vi "Write Websocket Data.vi"(6 "timeout ms (5000)":i32=500, 7 "Websocket Client Handler in":refnum<class "Websocket Client Handler.lvclass">, 8 "error in (no error)":errorcluster, 11 "Data":string) -> (0 "error out":errorcluster, 5 "Websocket Client Handler out":refnum<class "Websocket Client Handler.lvclass">)   [LabVIEW 2016, in "Stream Mediator.lvlib" / "Websocket Client Handler.lvclass"]
doc: "--\nCopyright © 2017 Composed SystemsI All rights reserved.\n\nAuthor: Jon McBee <jon.mcbee@composed.io>\n\nThis library is provided \"AS IS\" ,WITHOUT WARRANTIES OR\nCONDITIONS OF ANY KIND, either express or implied.\n\nComposed Systems -- composed.io\n\nStream 0.0.1.1\nJon McBee - Composed Systems\nCopyright (c) 2017, Composed Systems"
uses:
  <userlib>/Composed Systems/Stream/Mediator/Classes/Websocket Client Handler Actor/Websocket Client Handler/Websocket Client Handler.lvclass
  <userlib>/Composed Systems/Stream/Mediator/Classes/Websocket Client Handler Actor/Websocket Client Handler/Websocket Client Handler.lvclass/Websocket Client Handler.ctl
  <vilib>/MediaMongrels Ltd/WebSockets/WebSockets/WebSockets.lvlib
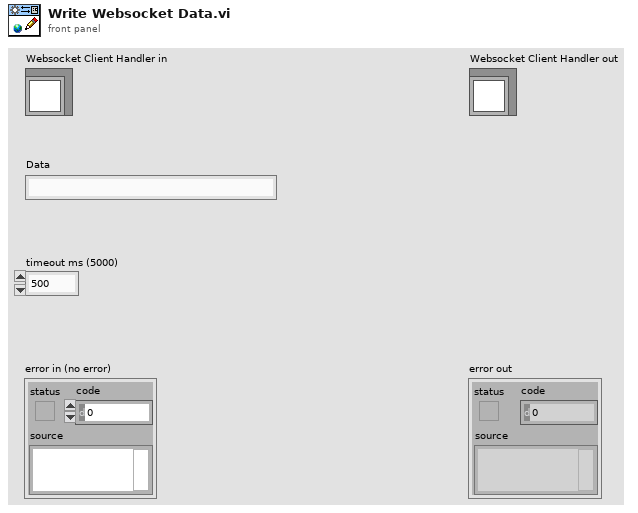
[diagram p1: front panel]
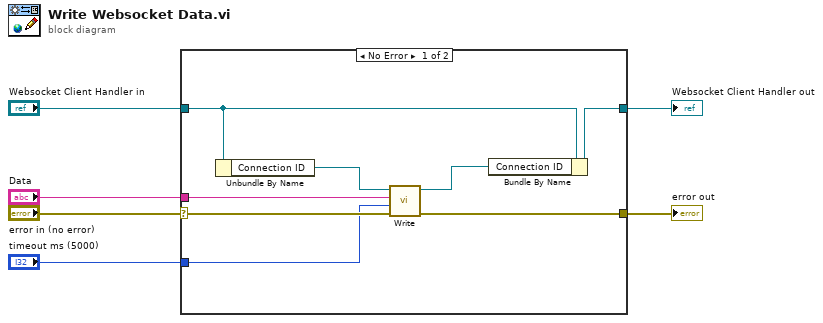
[diagram p0: block diagram]
diagram:
  n1 = case shown="No Error" "error in (no error)" {
    selector: "error in (no error)" -> [w14 w16]
    tunnel: [w13 w16] -> w5
    tunnel: [w7 w15] -> w3
    tunnel: "Websocket Client Handler in" -> [w8 w15]
    tunnel: "Data" -> [w12 _]
    tunnel: "timeout ms (5000)" -> [w11 _]
    frame No Error {
      n2 = Unbundle By Name(w8) -> ("Connection ID"=w10:refnum<k5>)
      n3 = call <vilib>:"Write.vi"("error in (no error)"=w14, "timeout ms (5000)"=w11, "Data"=w12, "WebSocket Connection in"=w10) -> ("error out"=w13:errorcluster, "WebSocket Connection out"=w9:refnum<k5>)  [unwired: 6 in]
      n4 = Bundle By Name(cluster=w8, "Connection ID"=w9) -> (w7:refnum<class "Websocket Client Handler.lvclass">)
    }
    frame Error {
    }
  }
  "error out" <- w5
  "Websocket Client Handler out" <- w3
